vi "Error Converter (ErrCode or Status).vi"(7 "path override":path, 8 "error in (no error)":errorcluster, 11 "error code":i32) -> (0 "error out":errorcluster)   [LabVIEW 2025, in "libzmq-v143-mt-4_3_6.lvlib"]
uses:
  libzmq-v143-mt-4_3_6.lvlib
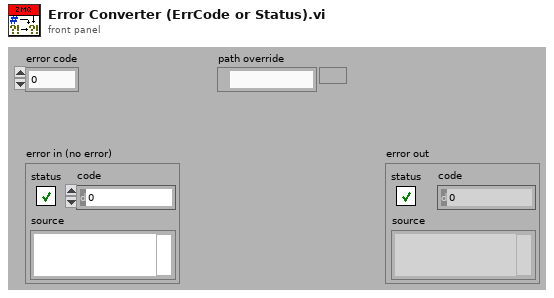
[diagram p1: front panel]
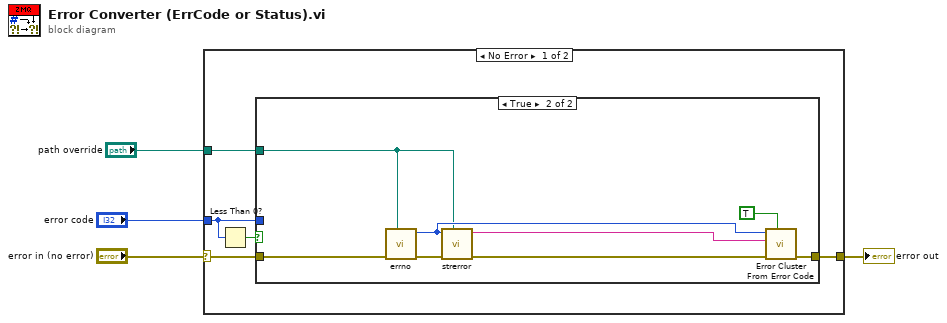
[diagram p0: block diagram]
diagram:
  n1 = case shown="No Error" "error in (no error)" {
    selector: "error in (no error)" -> [w8 w19]
    tunnel: [w6 w19] -> w3
    tunnel: "error code" -> [w7 _]
    tunnel: "path override" -> [w5 _]
    frame No Error {
      n2 = Less Than 0?(x=w7) -> (x < 0?=w9:bool)
      n3 = case shown="True" w9 {
        tunnel: w8 -> [w10 w13]
        tunnel: w7 -> [_ _]
        tunnel: [w10 w18] -> w6
        tunnel: w5 -> [_ w11]
        frame False {
        }
        frame True {
          n4 = call "errno.vi"("path override"=w11, "error in (no error)"=w13) -> ("error out"=w16:errorcluster, "function return"=w15:i32)  [unwired: 8 in]
          n5 = call "strerror.vi"("path override"=w11, "error in (no error)"=w16, "errnum_"=w15) -> ("error out"=w12:errorcluster, "function return"=w14:string)  [unwired: 7 in]
          n6 = call <vilib>:"Error Cluster From Error Code.vi"("show call chain? (False)"=TRUE, "error in (no error)"=w12, "error message (\"\")"=w14, "error code (0)"=w15) -> ("error out"=w18:errorcluster)  [unwired: 5 in]
        }
      }
    }
    frame Error {
    }
  }
  "error out" <- w3
